vi "Main.vi"() -> ()   [LabVIEW 2017, in "Server.lvlib"]
doc: "This is the Main VI of the Dashboard Server Application. It consists of a QMH with several Loops. See the loop descriptions for details."
uses:
  Server.lvlib
  TypeDefs/SR List.ctl
  TypeDefs/SR Data.ctl
  TypeDefs/ClientList.ctl
  TypeDefs/ClientData.ctl
  SubLibs/Message Queue/EnqueueMessage(Single).vi
  <vilib>/Utility/error.llb/Error Cluster From Error Code.vi
  <vilib>/ErrorRing/Error Ring.xnode
  SubLibs/Message Queue/Message Queue.lvlib
  SubLibs/ErrorLogger/ErrorLogger.lvlib
  SubLibs/Oracle/Oracle.lvlib
  SubLibs/WebServiceCommunication/WebServiceCommunication.lvlib
panel:
  out "ClientList":T1
  in  "GetCurrentClients":bool
  out "CurrentSRs":T3 {"SR#" format="%#_10g"}
  in  "Exit":bool
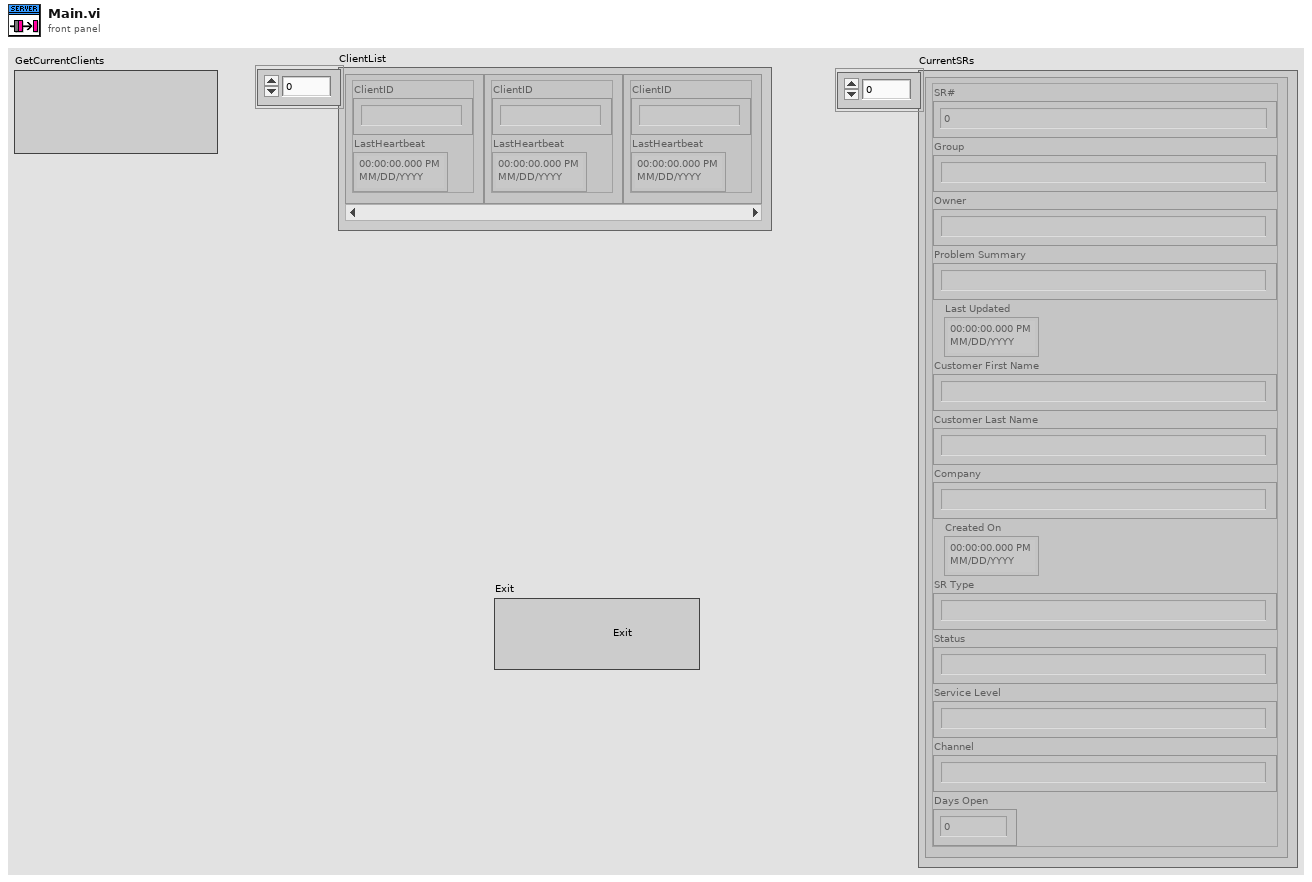
[diagram p1: front panel]
types:
  T1 = typedef "Server.lvlib/ClientList.ctl" = T2[]
  T2 = typedef "Server.lvlib/ClientData.ctl" = cluster{"ClientID":string, "LastHeartbeat":timestamp}
  T3 = typedef "Server.lvlib/SR List.ctl" = T4[]
  T4 = typedef "Server.lvlib/SR Data.ctl" = cluster{"SR#":dbl, "Group":string, "Owner":string, "Problem Summary":string, "Last Updated":timestamp, "Customer First Name":string, "Customer Last Name":string, "Company":string, "Created On":timestamp, "SR Type":string, "Status":string, "Service Level":string, "Channel":string, "Days Open":dbl}
  T5 = typedef "Server.lvlib/Message Queue.lvlib/CommReferences.ctl" = cluster{"MHL":refnum<queue>, "Error":refnum<queue>, "EventReg":refnum<event-registration>, "Event":refnum<user-event>, "UI":refnum<queue>, "WebServ":refnum<queue>, "Oracle":refnum<queue>}
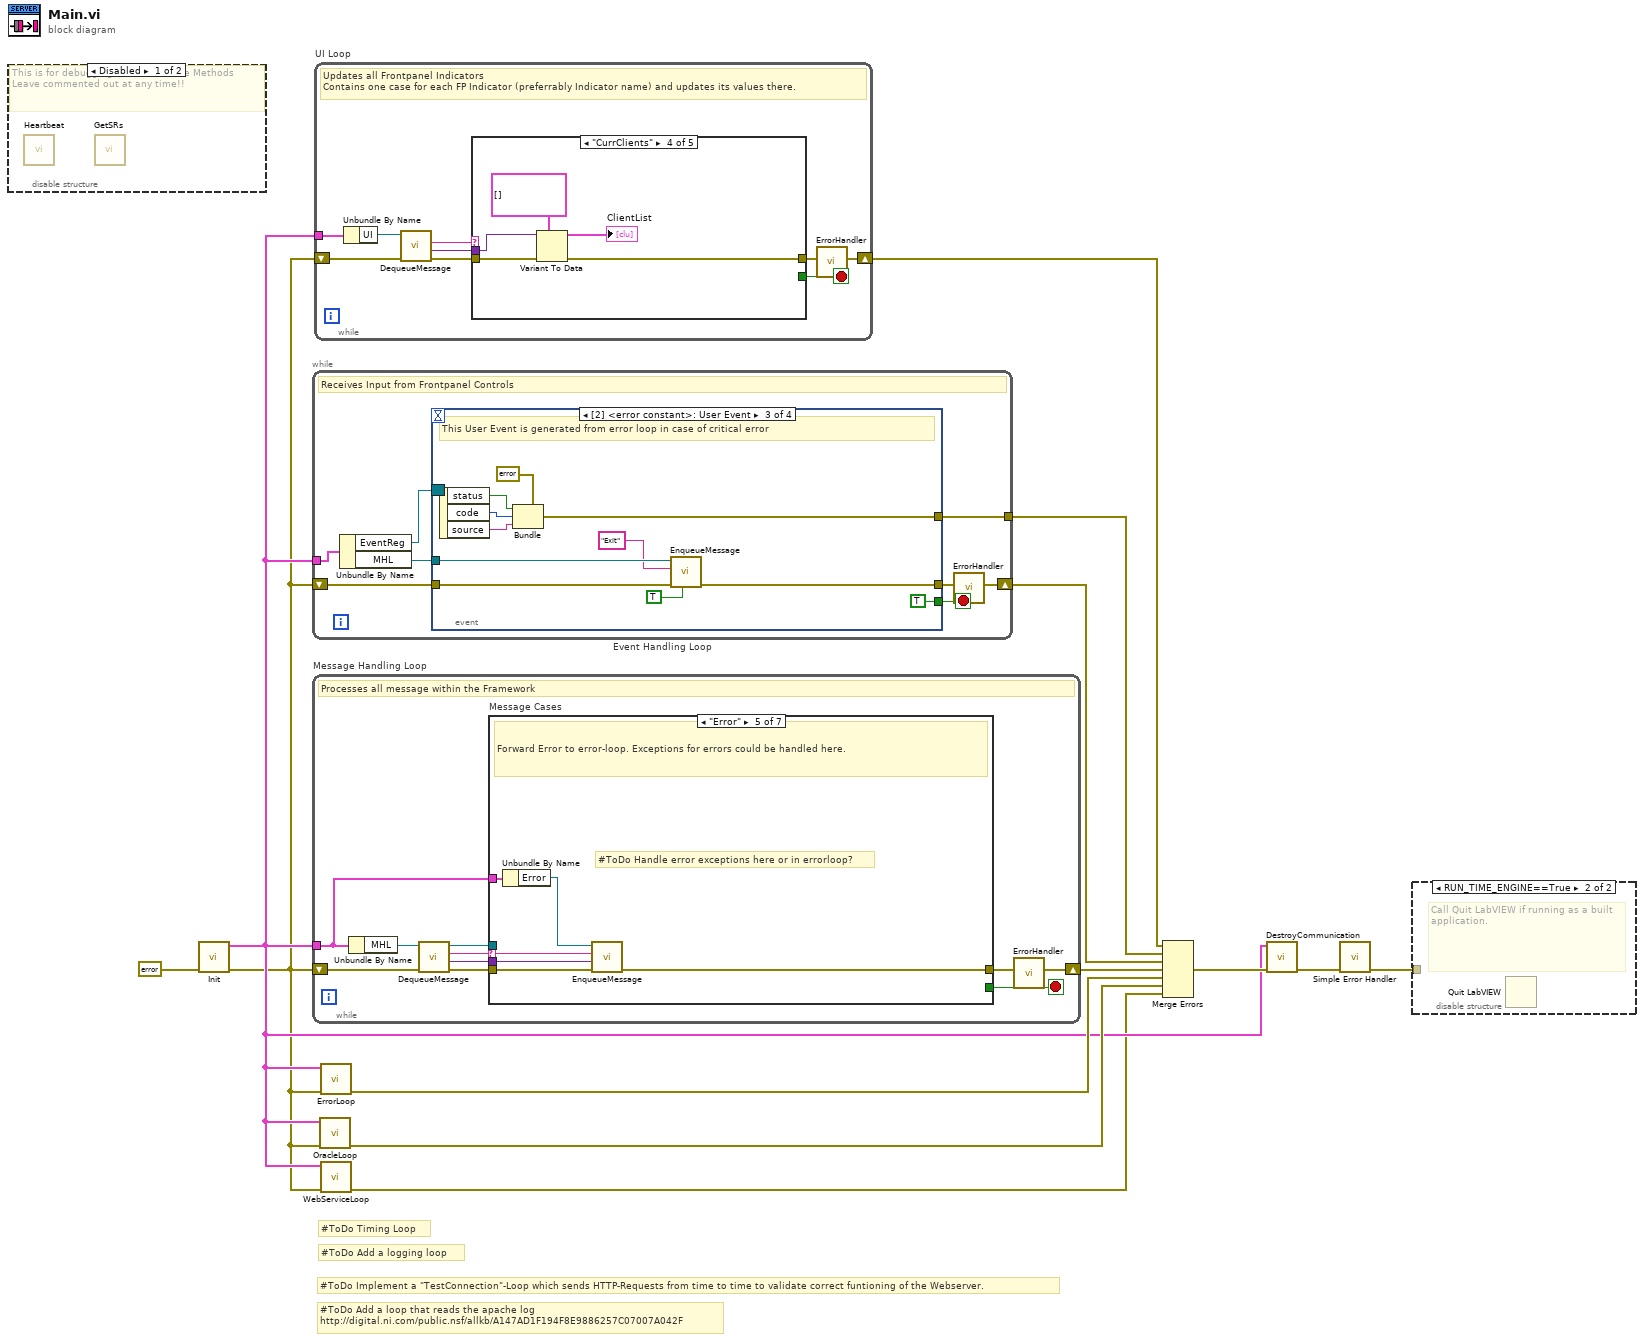
[diagram p0: block diagram]
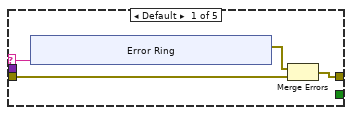
[diagram p3: hidden frame]
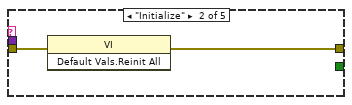
[diagram p4: hidden frame]
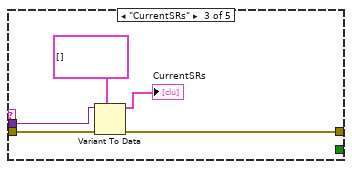
[diagram p5: hidden frame]
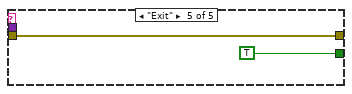
[diagram p6: hidden frame]
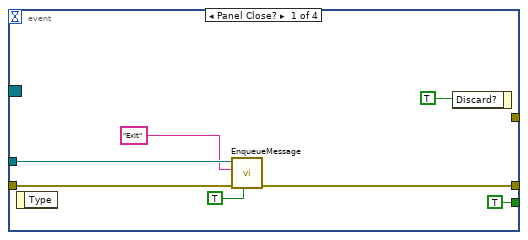
[diagram p8: hidden frame]
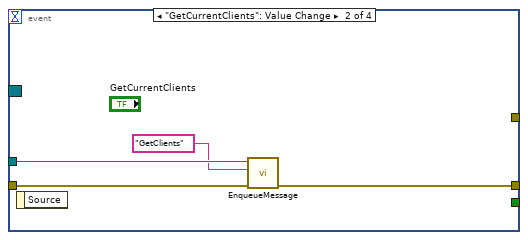
[diagram p9: hidden frame]
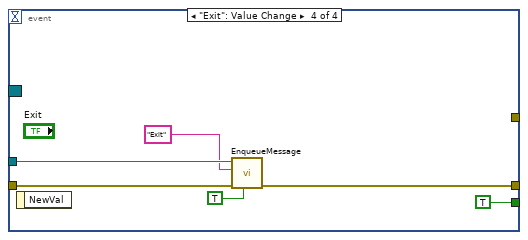
[diagram p10: hidden frame]
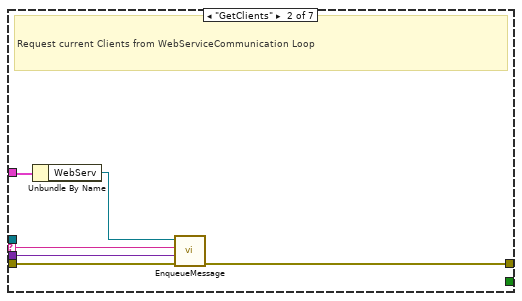
[diagram p12: hidden frame]
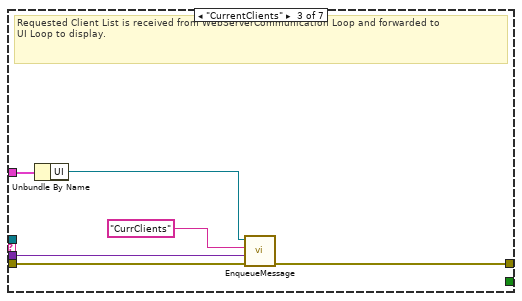
[diagram p13: hidden frame]
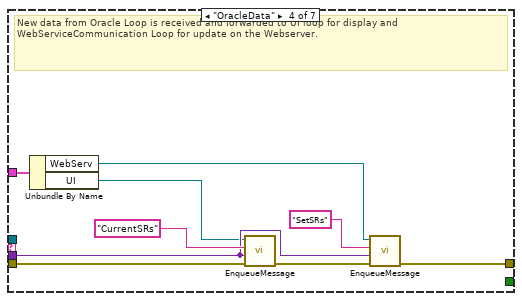
[diagram p14: hidden frame]
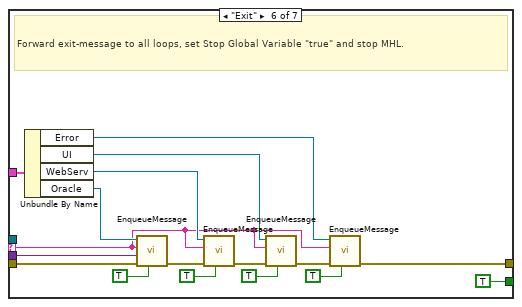
[diagram p15: hidden frame]
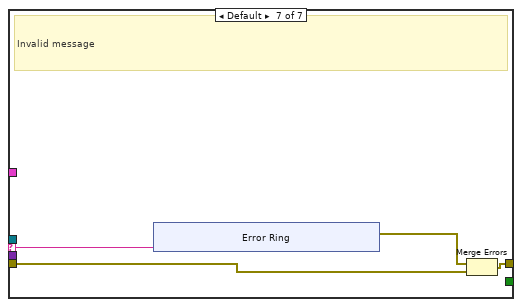
[diagram p16: hidden frame]
diagram:
  # "#ToDo Timing Loop"
  # "#ToDo Add a loop that reads the apache log\nhttp://digital.ni.com/public.nsf/allkb/A147AD1F194F8E9886257C07007A042F"
  # "#ToDo Add a logging loop"
  # "#ToDo Implement a \"TestConnection\"-Loop which sends HTTP-Requests from time to time to validate correct funtioning of the Webserver."
  n1 = disable-structure shown="Disabled" {
    frame Disabled {
      # "This is for debugging the Webservice Methods\nLeave commented out at any time!!"
      n2 = call "Heartbeat.vi"() -> ()  [unwired: 12 in]
      n3 = call "GetSRs.vi"() -> ()  [unwired: 11 in, 1 out]
    }
    frame Enabled {
    }
  }
  n4 = call "Init.vi"("error in (no error)"=errorcluster {"status"=FALSE, "code"=0, "source"=""}) -> ("error out"=w1:errorcluster, "Message Queues out"=w4:T5)  [unwired: 9 in]
  n5 = while "Event Handling Loop" {
    tunnel: w4 -> [w21]
    shift-right: [w15] -> w12
    shift-left: w1 -> [w18]
    tunnel: [w16] -> w9
    stop <- w14 stop-if-true
    # "Receives Input from Frontpanel Controls"
    n6 = Unbundle By Name(w21) -> ("EventReg"=w19:refnum<event-registration>, "MHL"=w20:refnum<queue>)
    n7 = event shown="[2] <error constant>: User Event" {
      selector: w19 -> [_ _ _ _]
      dyn-events: _ -> [_ _ _ _]
      timeout: _ -> [_ _ _ _]
      tunnel: w20 -> [w27 w30 w36 w49]
      tunnel: [w26 w31 w37 w48] -> w17
      tunnel: w18 -> [w23 w32 w43 w44]
      tunnel: [_ _ w38 _] -> w16
      tunnel: [TRUE ("Priority Message? (F)") _ TRUE ("Priority Message? (F)") TRUE ("Priority Message? (F)")] -> w14
      event Panel Close? {
        n8 = event-data() -> ()  [unwired: 1 in, 1 out]
        n9 = call-poly "EnqueueMessage.vi"("Priority Message? (F)"=TRUE, "error in (no error)"=w23, "Message"="Exit", "Message Queue"=w27) -> ("error out"=w26:errorcluster)  [unwired: 6 in, 1 out]
        n10 = event-data("Discard?"=TRUE) -> ()  [unwired: 1 in, 1 out]
      }
      event "GetCurrentClients": Value Change {
        n11 = event-data() -> ()  [unwired: 1 in, 1 out]
        n12 = call-poly "EnqueueMessage.vi"("error in (no error)"=w32, "Message"="GetClients", "Message Queue"=w30) -> ("error out"=w31:errorcluster)  [unwired: 7 in, 1 out]
      }
      event User Event {
        # "This User Event is generated from error loop in case of critical error"
        n13 = event-data() -> ("status"=w41:bool, "code"=w40:i32, "source"=w39:string)  [unwired: 1 in]
        n14 = Bundle(cluster=errorcluster {"status"=FALSE, "code"=0, "source"=""} ("error constant"), "status"=w41, "code"=w40, "source"=w39) -> (w38:errorcluster)
        n15 = call-poly "EnqueueMessage.vi"("Priority Message? (F)"=TRUE, "error in (no error)"=w43, "Message"="Exit", "Message Queue"=w36) -> ("error out"=w37:errorcluster)  [unwired: 6 in, 1 out]
      }
      event "Exit": Value Change {
        n16 = event-data() -> ()  [unwired: 1 in, 1 out]
        n17 = call-poly "EnqueueMessage.vi"("Priority Message? (F)"=TRUE, "error in (no error)"=w44, "Message"="Exit", "Message Queue"=w49) -> ("error out"=w48:errorcluster)  [unwired: 6 in, 1 out]
      }
    }
    n18 = call "ErrorHandler.vi"("Error In"=w17) -> ("Error Out"=w15:errorcluster)  [unwired: 10 in]
  }
  n19 = while "Message Handling Loop" {
    tunnel: w4 -> [w50]
    shift-right: [w51] -> w13
    shift-left: w1 -> [w58]
    stop <- w59 stop-if-true
    # "Processes all message within the Framework"
    n20 = Unbundle By Name(w50) -> ("MHL"=w53:refnum<queue>)
    n21 = call "DequeueMessage.vi"("error in (no error)"=w58, "Message Queue"=w53) -> ("error out"=w57:errorcluster, "Message Data"=w55:variant, "Message"=w56:string, "dup Message Queue"=w54:refnum<queue>)  [unwired: 5 in, 1 out]
    n22 = case "Message Cases" shown="\"Error\"" w56 {
      selector: w56 -> [_ w64 _ _ w84 w90 w106]
      tunnel: w54 -> [_ _ _ _ _ _ _]
      tunnel: w57 -> [w60 w66 w72 w80 w86 w102 w104]
      tunnel: [w60 w65 w71 w79 w85 w95 w105] -> w52
      tunnel: [_ _ _ _ _ TRUE _] -> w59
      tunnel: w55 -> [_ w63 w70 w77 w83 w101 _]
      tunnel: w50 -> [_ w62 w68 w75 w82 w96 _]
      frame "Initialize" {
        # "Send Initial Values to necessary loops"
      }
      frame "GetClients" {
        # "Request current Clients from WebServiceCommunication Loop"
        n23 = Unbundle By Name(w62) -> ("WebServ"=w61:refnum<queue>)
        n24 = call-poly "EnqueueMessage.vi"("error in (no error)"=w66, "Message Data"=w63, "Message"=w64, "Message Queue"=w61) -> ("error out"=w65:errorcluster)  [unwired: 6 in, 1 out]
      }
      frame "CurrentClients" {
        # "Requested Client List is received from WebServerCommunication Loop and forwarded to \nUI Loop to display."
        n25 = Unbundle By Name(w68) -> ("UI"=w67:refnum<queue>)
        n26 = call-poly "EnqueueMessage.vi"("error in (no error)"=w72, "Message Data"=w70, "Message"="CurrClients", "Message Queue"=w67) -> ("error out"=w71:errorcluster)  [unwired: 6 in, 1 out]
      }
      frame "OracleData" {
        # "New data from Oracle Loop is received and forwarded to UI loop for display and WebServiceCommunication Loop for update on the Webserver."
        n27 = Unbundle By Name(w75) -> ("WebServ"=w73:refnum<queue>, "UI"=w74:refnum<queue>)
        n28 = call-poly "EnqueueMessage.vi"("error in (no error)"=w80, "Message Data"=w77, "Message"="CurrentSRs", "Message Queue"=w74) -> ("error out"=w79:errorcluster)  [unwired: 6 in, 1 out]
        n29 = call-poly "EnqueueMessage.vi"("Message Data"=w77, "Message"="SetSRs", "Message Queue"=w73) -> ()  [unwired: 7 in, 2 out]
      }
      frame "Error" {
        # "#ToDo Handle error exceptions here or in errorloop?"
        # "Forward Error to error-loop. Exceptions for errors could be handled here."
        n30 = Unbundle By Name(w82) -> ("Error"=w81:refnum<queue>)
        n31 = call-poly "EnqueueMessage.vi"("error in (no error)"=w86, "Message Data"=w83, "Message"=w84, "Message Queue"=w81) -> ("error out"=w85:errorcluster)  [unwired: 6 in, 1 out]
      }
      frame "Exit" {
        # "Forward exit-message to all loops, set Stop Global Variable \"true\" and stop MHL."
        n32 = Unbundle By Name(w96) -> ("Error"=w91:refnum<queue>, "UI"=w92:refnum<queue>, "WebServ"=w93:refnum<queue>, "Oracle"=w94:refnum<queue>)
        n33 = call-poly "EnqueueMessage.vi"("Priority Message? (F)"=TRUE, "error in (no error)"=w102, "Message Data"=w101, "Message"=w90, "Message Queue"=w94) -> ("error out"=w99:errorcluster)  [unwired: 5 in, 1 out]
        n34 = call-poly "EnqueueMessage.vi"("Priority Message? (F)"=TRUE, "error in (no error)"=w99, "Message"=w90, "Message Queue"=w93) -> ("error out"=w98:errorcluster)  [unwired: 6 in, 1 out]
        n35 = call-poly "EnqueueMessage.vi"("Priority Message? (F)"=TRUE, "error in (no error)"=w98, "Message"=w90, "Message Queue"=w92) -> ("error out"=w97:errorcluster)  [unwired: 6 in, 1 out]
        n36 = call-poly "EnqueueMessage.vi"("Priority Message? (F)"=TRUE, "error in (no error)"=w97, "Message"=w90, "Message Queue"=w91) -> ("error out"=w95:errorcluster)  [unwired: 6 in, 1 out]
      }
      frame Default {
        # "Invalid message"
        n37 = xnode "Error Ring"("parameter 0"=w106) -> ("error out"=w107:errorcluster)
        n38 = Merge Errors(w107, w104) -> (w105:errorcluster)
      }
    }
    n39 = call "ErrorHandler.vi"("Error In"=w52) -> ("Error Out"=w51:errorcluster)  [unwired: 10 in]
  }
  n40 = while "UI Loop" {
    shift-right: [w122] -> w3
    shift-left: w1 -> [w123]
    tunnel: w4 -> [w121]
    stop <- w115 stop-if-true
    # "Updates all Frontpanel Indicators\nContains one case for each FP Indicator (preferrably Indicator name) and updates its values there."
    n41 = Unbundle By Name(w121) -> ("UI"=w120:refnum<queue>)
    n42 = call "DequeueMessage.vi"("error in (no error)"=w123, "Message Queue"=w120) -> ("error out"=w118:errorcluster, "Message Data"=w116:variant, "Message"=w119:string)  [unwired: 5 in, 2 out]
    n43 = case shown="\"CurrClients\"" w119 {
      selector: w119 -> [w126 _ _ _ _]
      tunnel: [w125 w135 w140 w145 w148] -> w117
      tunnel: w118 -> [w127 w136 w141 w146 w148]
      tunnel: w116 -> [_ _ w137 w144 _]
      tunnel: [_ _ _ _ TRUE] -> w115
      frame Default {
        n44 = xnode "Error Ring"("parameter 0"=w126) -> ("error out"=w124:errorcluster)
        n45 = Merge Errors(w124, w127) -> (w125:errorcluster)
      }
      frame "Initialize" {
        n46 = invoke class="VI" method="Default Vals.Reinit All"(error in=w136) -> (error out=w135:errorcluster)  [unwired: 2 in, 2 out]
      }
      frame "CurrentSRs" {
        n47 = Variant To Data(error in=w141, type=T3 [] ("CurrentSRs"), Variant=w137) -> (data=→"CurrentSRs":T3, error out=w140:errorcluster)
      }
      frame "CurrClients" {
        n48 = Variant To Data(error in=w146, type=T1 [] ("ClientList"), Variant=w144) -> (data=→"ClientList":T1, error out=w145:errorcluster)
      }
      frame "Exit" {
      }
    }
    n49 = call "ErrorHandler.vi"("Error In"=w117) -> ("Error Out"=w122:errorcluster)  [unwired: 10 in]
  }
  n50 = call "OracleLoop.vi"("Error In"=w1, "Message Queues"=w4) -> ("Error Out"=w5:errorcluster)  [unwired: 9 in]
  n51 = call "ErrorLoop.vi"("Error In"=w1, "Message Queues"=w4) -> ("Error Out"=w7:errorcluster)  [unwired: 9 in]
  n52 = call "WebServiceLoop.vi"("Error In"=w1, "Message Queues"=w4) -> ("Error Out"=w2:errorcluster)  [unwired: 9 in]
  n53 = Merge Errors(w3, w9, w12, w13, w7, w5, w2) -> (w11:errorcluster)
  n54 = call "DestroyCommunication.vi"("error in (no error)"=w11, "Message Queues out"=w4) -> ("error out"=w8:errorcluster)  [unwired: 9 in]
  n55 = call <vilib>:"Simple Error Handler.vi"("error in (no error)"=w8) -> ("error out"=w6:errorcluster)  [unwired: 4 in, 4 out]
  n56 = disable-structure shown="RUN_TIME_ENGINE==True" {
    disable-tunnel: w6 -> [_ _]
    frame condition #0 (active) {
    }
    frame condition #1 {
      # "Call Quit LabVIEW if running as a built application."
      n57 = Quit LabVIEW() -> ()  [unwired: 1 in]
    }
  }
